vi "ex_SaveFileCheckNameTDMS.vi"(4 "file exists?":bool, 5 "overwrite_mode_multi":T3(ring)=enum."overwrite & backup", 6 "multi_file":bool, 7 "overwrite_mode":T4(ring), 8 "error in (no error)":errorcluster, 10 "file params in":T1={"delimiter"="\t", "origin time"=timestamp(0 s since 1904-01-01), "Flags"={"include col headings?"=TRUE, "x_columns"=0, "col headings always?"=TRUE, "time preference"=0, "hide col headings"=FALSE}, "Decimal Separator"=""} {"Flags"."time preference" items=["Absolute", "Relative"]; "Flags"."x_columns" items=["None", "One", "Multiple"]; "origin time" format="%<%X\n%x>T"}, 11 "file path":path) -> (0 "error out":errorcluster, 1 "tdms file out":refnum<k34>, 2 "file params out":T1={"delimiter"="\t", "origin time"=timestamp(0 s since 1904-01-01), "Flags"={"include col headings?"=TRUE, "x_columns"=0, "col headings always?"=TRUE, "time preference"=0, "hide col headings"=FALSE}, "Decimal Separator"=""} {"Flags"."time preference" items=["Absolute", "Relative"]; "Flags"."x_columns" items=["None", "One", "Multiple"]; "origin time" format="%<%X\n%x>T"}, 3 "file path out":path)   [LabVIEW 2020]
uses:
  <vilib>/express/express output/ExFileWriteBlock.llb/ex_WriteFileParams.ctl
  <vilib>/express/express input/ExFileReadBlock.llb/ex_ReadFileParams.ctl
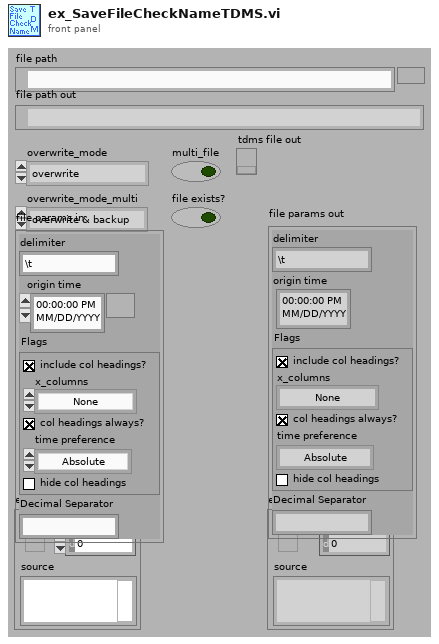
[diagram p1: front panel]
types:
  T1 = typedef "ex_WriteFileParams.ctl" = cluster{"delimiter":string, "origin time":timestamp, "Flags":T2, "Decimal Separator":string}
  T2 = typedef "ex_ReadFileParams.ctl" = cluster{"include col headings?":bool, "x_columns":u16, "col headings always?":bool, "time preference":u16, "hide col headings":bool}
  T3 = enum16{"overwrite", "overwrite & backup", "next avail"}
  T4 = enum16{"overwrite", "overwrite & backup", "append", "next avail"}
  T5 = enum16{"open", "open or create", "create or replace", "create", "open (read-only)"}
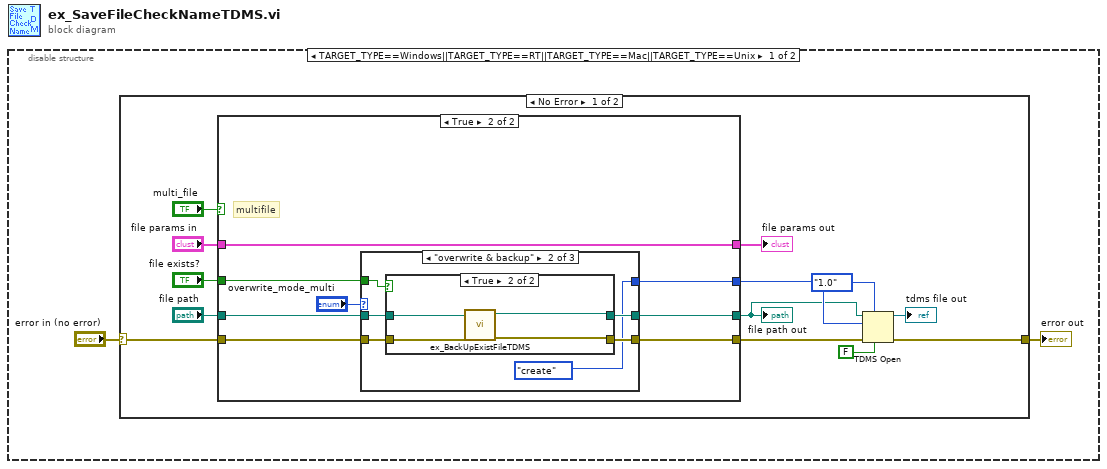
[diagram p0: block diagram]
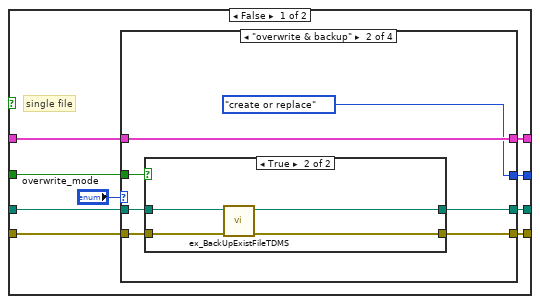
[diagram p2: hidden frame]
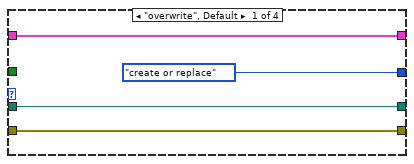
[diagram p3: hidden frame]
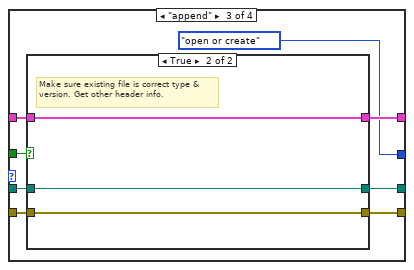
[diagram p5: hidden frame]
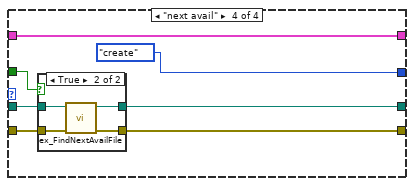
[diagram p7: hidden frame]
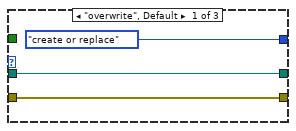
[diagram p9: hidden frame]
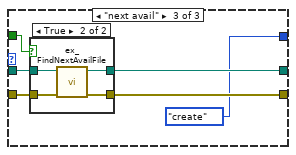
[diagram p11: hidden frame]
diagram:
  n1 = disable-structure shown="TARGET_TYPE==Windows||TARGET_TYPE==RT||TARGET_TYPE==Mac||TARGET_TYPE==Unix" {
    frame condition #0 (active) {
      n2 = case shown="No Error" "error in (no error)" {
        selector: "error in (no error)" -> [w12 w104]
        tunnel: [w8 w104] -> w2
        frame No Error {
          n3 = case shown="True" "multi_file" {
            tunnel: [w23 w75] -> w7
            tunnel: "file path" -> [w18 w74]
            tunnel: [w20 w69] -> w6
            tunnel: [w19 w72] -> w9
            tunnel: "file exists?" -> [w22 w71]
            tunnel: w12 -> [w21 w73]
            tunnel: [w16 w70] -> w10
            tunnel: "file params in" -> [w17 w70]
            frame False {
              # "single file"
              n4 = case shown="\"overwrite & backup\"" "overwrite_mode" {
                tunnel: [T5."create or replace" ("operation") T5."create or replace" ("operation") T5."open or create" ("operation") T5."create" ("operation")] -> w23
                tunnel: w22 -> [_ w31 w48 w58]
                tunnel: w18 -> [w28 w33 w44 w62]
                tunnel: w21 -> [w27 w32 w49 w59]
                tunnel: [w28 w35 w43 w60] -> w20
                tunnel: [w27 w34 w47 w61] -> w19
                tunnel: [w26 w30 w46 w57] -> w16
                tunnel: w17 -> [w26 w30 w45 w57]
                frame "overwrite", Default {
                }
                frame "overwrite & backup" {
                  n5 = case shown="True" w31 {
                    tunnel: w33 -> [w36 w41]
                    tunnel: w32 -> [w37 w40]
                    tunnel: [w36 w38] -> w35
                    tunnel: [w37 w39] -> w34
                    frame False {
                      # "File doesn't exist-- do nothing"
                    }
                    frame True {
                      n6 = call <vilib>:"ex_BackUpExistFileTDMS.vi"("error in"=w40, "file path"=w41) -> ("error out"=w39:errorcluster, "dup file path"=w38:path)  [unwired: 8 out]
                    }
                  }
                }
                frame "append" {
                  n7 = case shown="True" w48 {
                    tunnel: w49 -> [w51 w53]
                    tunnel: w44 -> [w50 w55]
                    tunnel: [w51 w53] -> w47
                    tunnel: [w52 w54] -> w46
                    tunnel: w45 -> [w52 w54]
                    tunnel: [w50 w55] -> w43
                    frame False {
                    }
                    frame True {
                      # "Make sure existing file is correct type & version. Get other header info."
                    }
                  }
                }
                frame "next avail" {
                  n8 = case shown="True" w58 {
                    tunnel: w62 -> [w64 w68]
                    tunnel: [w63 w67] -> w61
                    tunnel: [w64 w66] -> w60
                    tunnel: w59 -> [w63 w65]
                    frame False {
                    }
                    frame True {
                      n9 = call <vilib>:"ex_FindNextAvailFile.vi"("error in"=w65, "desired file path"=w68) -> ("error out"=w67:errorcluster, "next avail file path"=w66:path)  [unwired: 8 out]
                    }
                  }
                }
              }
            }
            frame True {
              # "multifile"
              n10 = case shown="\"overwrite & backup\"" "overwrite_mode_multi" {
                tunnel: [T5."create or replace" ("operation") T5."create" ("operation") T5."create" ("operation")] -> w75
                tunnel: w74 -> [w79 w85 w95]
                tunnel: w73 -> [w78 w84 w94]
                tunnel: [w79 w82 w97] -> w69
                tunnel: [w78 w81 w96] -> w72
                tunnel: w71 -> [_ w83 w93]
                frame "overwrite", Default {
                }
                frame "overwrite & backup" {
                  n11 = case shown="True" w83 {
                    tunnel: w85 -> [w86 w91]
                    tunnel: w84 -> [w87 w90]
                    tunnel: [w86 w89] -> w82
                    tunnel: [w87 w88] -> w81
                    frame False {
                      # "File doesn't exist-- do nothing"
                    }
                    frame True {
                      n12 = call <vilib>:"ex_BackUpExistFileTDMS.vi"("error in"=w90, "file path"=w91) -> ("error out"=w88:errorcluster, "dup file path"=w89:path)  [unwired: 8 out]
                    }
                  }
                }
                frame "next avail" {
                  n13 = case shown="True" w93 {
                    tunnel: w95 -> [w99 w103]
                    tunnel: [w98 w102] -> w96
                    tunnel: [w99 w101] -> w97
                    tunnel: w94 -> [w98 w100]
                    frame False {
                    }
                    frame True {
                      n14 = call <vilib>:"ex_FindNextAvailFile.vi"("error in"=w100, "desired file path"=w103) -> ("error out"=w102:errorcluster, "next avail file path"=w101:path)  [unwired: 8 out]
                    }
                  }
                }
              }
            }
          }
          "file path out" <- w6
          "file params out" <- w10
          n15 = TDMS Open(6:FALSE ("disable buffering? (T)"), 7:enum16{"1.0", "2.0"}."1.0" ("file format version (2.0)"), 8:w9, 10:w7, 11:w6) -> (0:w8:errorcluster, 3:→"tdms file out":refnum<k34>)  [unwired: 2 in]
        }
        frame Error {
        }
      }
      "error out" <- w2
    }
    frame condition #1 {
    }
  }
